vi "SplineHelp_GetCubicSpline_Calc1.vi"(4 "Y-Initial-1":dbl, 6 "X-Initial-1":dbl, 8 "newWayPoints":T1[](array[typedef]) {"Y" format="%14.3f"; "X" format="%14.3f"}, 9 "dy-in":dbl[](array[numeric]), 11 "dx-in":dbl[](array[numeric])) -> (1 "dy-out":dbl[](array[numeric]), 3 "dx-out":dbl[](array[numeric]))   [LabVIEW 2019, in "Trajectory_Library.lvlib"]
doc: "Internal routine called by: SplineHelp_getCubicSplinesFromControlVectors.vi"
uses:
  Trajectory_Library.lvlib
  TypeDef/TRANSLATION2D.ctl
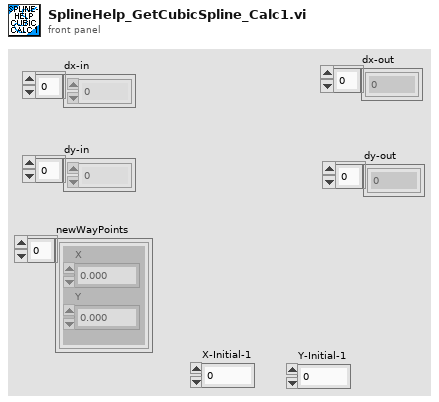
[diagram p1: front panel]
types:
  T1 = typedef "Trajectory_Library.lvlib/TRANSLATION2D.ctl" = cluster{"X":dbl, "Y":dbl}
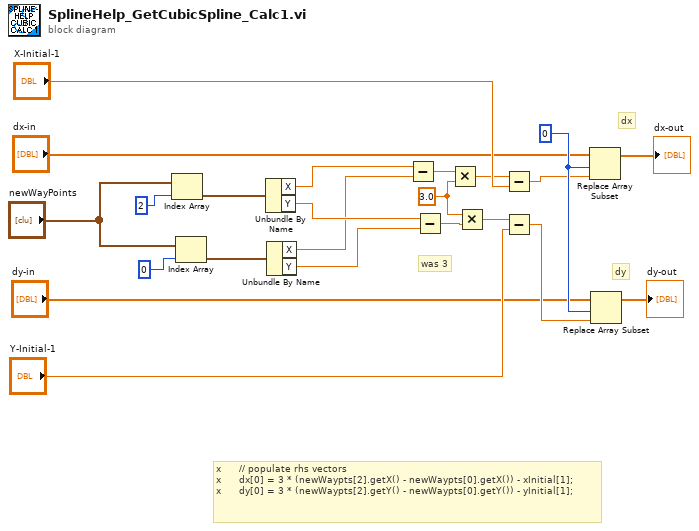
[diagram p0: block diagram]
diagram:
  w22 = 0 ("index")
  w12 = 3.0
  # "was 3"
  # "x      // populate rhs vectors\nx      dx[0] = 3 * (newWaypts[2].getX() - newWaypts[0].getX()) - xInitial[1];\nx      dy[0] = 3 * (newWaypts[2].getY() - newWaypts[0].getY()) - yInitial[1];"
  # "dy"
  # "dx"
  n1 = Index Array(array="newWayPoints", index=2) -> (element=w5:T1)
  n2 = Index Array(array="newWayPoints", index=0) -> (element=w1:T1)
  n3 = Unbundle By Name(w5) -> ("X"=w6:dbl, "Y"=w8:dbl)
  n4 = Unbundle By Name(w1) -> ("X"=w7:dbl, "Y"=w9:dbl)
  n5 = Subtract(x=w6, y=w7) -> (x-y=w10:dbl)
  n6 = Subtract(x=w8, y=w9) -> (x-y=w11:dbl)
  n7 = Multiply(x=w10, y=w12) -> (x*y=w13:dbl)
  n8 = Multiply(x=w12, y=w11) -> (x*y=w14:dbl)
  n9 = Subtract(x=w13, y="X-Initial-1") -> (x-y=w21:dbl)
  n10 = Subtract(x=w14, y="Y-Initial-1") -> (x-y=w23:dbl)
  n11 = Replace Array Subset(array="dx-in", new element=w21, index=w22) -> (→"dx-out":dbl[])
  n12 = Replace Array Subset(array="dy-in", new element=w23, index=w22) -> (→"dy-out":dbl[])
